vi "Safety Check.vi"(9 "Temperature":string, 11 "RPMs":string) -> (3 "Safe?":bool)   [LabVIEW 2017]
doc: "<b>Description</b>\nThis VI checks the given RPM and Temperature to ensure that they are within a safe range.\n\n<b>Inputs</b>\nRPMs: The RPMs to be checked.\nTemperature: The temperature to be checked.\n\n<b>Outputs</b>\nSafe?: True if both the RPMs and temperature are in a safe range. False if either value is outside of the safety limits."
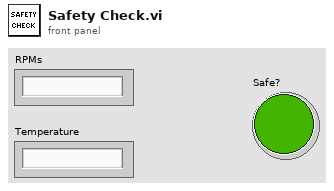
[diagram p1: front panel]
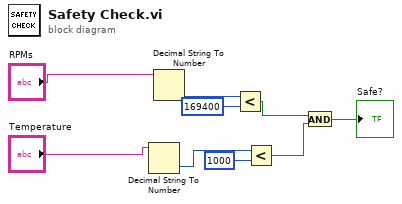
[diagram p0: block diagram]
diagram:
  n1 = Decimal String To Number(string="Temperature") -> (number=w5:i32)  [unwired: 2 in, 1 out]
  n2 = Decimal String To Number(string="RPMs") -> (number=w8:i32)  [unwired: 2 in, 1 out]
  n3 = Less?(x=w8, y=169400) -> (x < y?=w3:bool)
  n4 = Less?(x=w5, y=1000) -> (x < y?=w2:bool)
  n5 = And(x=w3, y=w2) -> (x .and. y?=→"Safe?":bool)
